vi "IntakeForTime.vi"() -> ()   [LabVIEW 2018]
uses:
  Framework/Robot Global Data.vi
panel:
  in  "NoWait":bool
  in  "Duration (s)":dbl
  in  "Speed":dbl
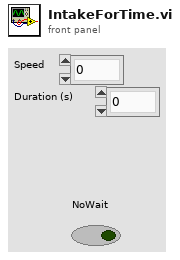
[diagram p1: front panel]
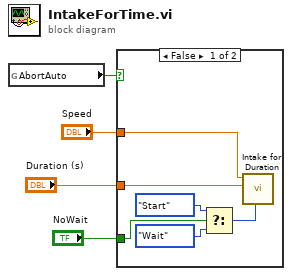
[diagram p0: block diagram]
diagram:
  n1 = global read "Robot Global Data.vi" "AbortAuto"() -> (w4:bool)
  n2 = case shown="False" w4 {
    tunnel: "NoWait" -> [w8 _]
    tunnel: "Speed" -> [w6 _]
    tunnel: "Duration (s)" -> [w5 _]
    frame False {
      n3 = Select(t=enum16{"Start", "Wait"}."Start", s=w8, f=enum16{"Start", "Wait"}."Wait" ("Synchronication")) -> (s? t:f=w7:enum16{"Start", "Wait"})
      n4 = call "Intake for Duration.vi"("Synchronization"=w7, "Duration (s)"=w5, "Speed"=w6) -> ()  [unwired: 8 in, 1 out]
    }
    frame True {
    }
  }
